vi "WMOLdll.vi"(8 "error in (no error)":errorcluster, 11 "z":dbl[](array[numeric])) -> (0 "error out":errorcluster, 2 "wmm out":dbl, 3 "z out":dbl[](array[numeric]))   [LabVIEW 2015]
doc: "function WMOL (x)\n\nmolecular weight for a mixture of specified composition\n\nINPUT:\nz -- composition array [array of mol frac]\n\nOUTPUTs:\nz -- composition array [array of mol frac]\nwmm -- molar mass [g/mol], a.k.a. \"molecular weight\""
uses:
  REFPROP.dll
panel:
  # "REFPROP-WMOL_dll.vi"
  # "void WMOLdll(double *z, double *wmm);"
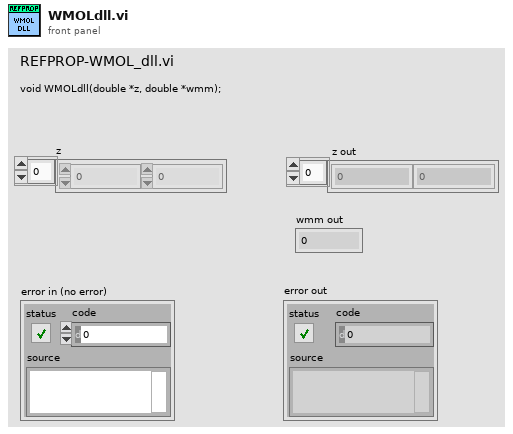
[diagram p1: front panel]
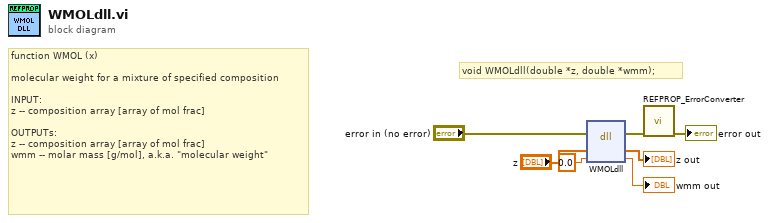
[diagram p0: block diagram]
diagram:
  # "function WMOL (x)\n\nmolecular weight for a mixture of specified composition\n\nINPUT:\nz -- composition array [array of mol frac]\n\nOUTPUTs:\nz -- composition array [array of mol frac]\nwmm -- molar mass [g/mol], a.k.a. \"molecular weight\""
  # "void WMOLdll(double *z, double *wmm);"
  n1 = dll-call lib="C:/Users/lauria/Desktop/REFPROP 10 LabVIEW Wrapper BETA/REFPROP/refprop.*" fn="WMOLdll"(error in="error in (no error)", "z"="z", "wmm"=0.0 ("wm")) -> (error out=w5:errorcluster, "z"=→"z out":dbl[], "wmm"=→"wmm out":dbl)  [unwired: 3 in, 1 out]
  n2 = call "REFPROP_ErrorConverter.vi"("error in (no error)"=w5) -> ("error out"=→"error out":errorcluster)  [unwired: 10 in]
